vi "Read Relation.vi"(11 "Base Teller in":refnum<class "Base Teller.lvclass">) -> (2 "Relation":T1)   [LabVIEW 2025, in "jettl.lvlib" / "Teller.lvlib" / "Base Teller.lvclass"]
uses:
  Base Teller.lvclass
  Relation.ctl
  Base Teller.lvclass/Base Teller.ctl
  jettl.lvlib
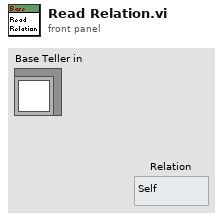
[diagram p1: front panel]
types:
  T1 = typedef "jettl.lvlib/Relation.ctl" = enum16{"Self", "Parent", "Child"}
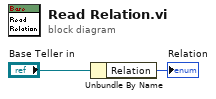
[diagram p0: block diagram]
diagram:
  n1 = Unbundle By Name("Base Teller in") -> ("Relation"=→"Relation":T1)
